vi "Event Handle Dispatcher.vi"(8 "error in (no error)":errorcluster, 11 "QTab Class in":refnum<class "QTab Class.lvclass">) -> (0 "error out":errorcluster)   [LabVIEW 2020, in "QTab.lvlib" / "QTab Class.lvclass"]
uses:
  QTab Class.lvclass
  Command.ctl
  QTab Class.lvclass/QTab Class.ctl
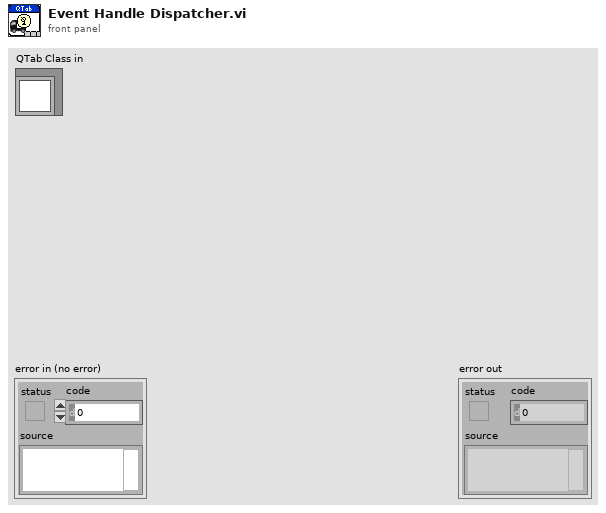
[diagram p1: front panel]
types:
  T1 = typedef "QTab.lvlib/QTab Class.lvclass/Command.ctl" = enum16{"Startup", "Add Page", "Close All Page", "Set Page Attribute", "Pop-out", "Merage", "Insert", "Stop"}
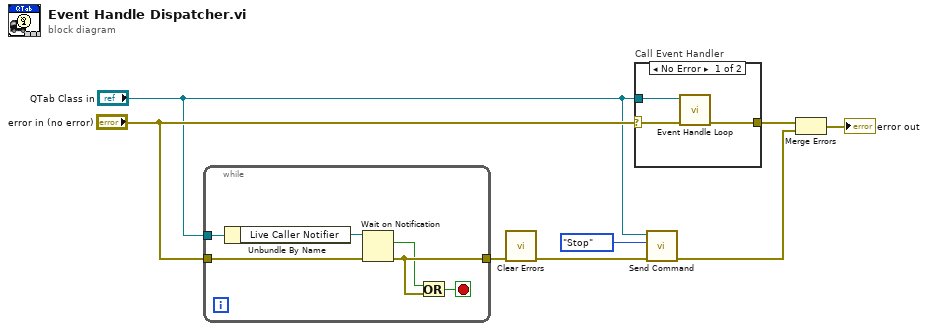
[diagram p0: block diagram]
diagram:
  n1 = while {
    tunnel: "QTab Class in" -> [w12]
    tunnel: "error in (no error)" -> [w13]
    tunnel: [w11] -> w7
    stop <- w9 stop-if-true
    n2 = Unbundle By Name(w12) -> ("Live Caller Notifier"=w14:refnum<notifier>)
    n3 = Wait on Notification(notifier=w14, error in (no error)=w13) -> (notification=w10:bool, error out=w11:errorcluster)  [unwired: 2 in, 2 out]
    n4 = Or(x=w10, y=w11) -> (x .or. y?=w9:bool)
  }
  n5 = call <vilib>:"Clear Errors.vi"("error in (no error)"=w7) -> ("error out"=w5:errorcluster)  [unwired: 5 in, 1 out]
  n6 = case "Call Event Handler" shown="No Error" "error in (no error)" {
    selector: "error in (no error)" -> [w17 w18]
    tunnel: [w15 w18] -> w8
    tunnel: "QTab Class in" -> [w16 _]
    frame No Error {
      n7 = call "Event Handle Loop.vi"("error in (no error)"=w17, "QTab Class in"=w16) -> ("error out"=w15:errorcluster)  [unwired: 8 in, 1 out]
    }
    frame Error {
    }
  }
  n8 = call "Send Command.vi"("error in (no error)"=w5, "Command"=Command."Stop", "QTab Class in"="QTab Class in") -> ("error out"=w2:errorcluster)  [unwired: 7 in, 1 out]
  n9 = Merge Errors(w8, w2) -> (→"error out":errorcluster)
